vi "DB Tools Move To Next Record.vi"   [LabVIEW 2013, in "NI_Database_API_64.lvlib"]
doc: "Moves the cursor to point to the next record in the recordset identified by the reference. Wire data to the reference input to determine the polymorphic instance to use or manually select the instance."
uses:
  NI_Database_API_64.lvlib
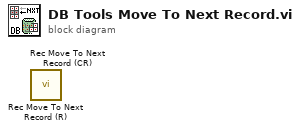
[diagram p0: block diagram]
diagram:
  n1 = call "Rec Move To Next Record (R).vi"() -> ()  [unwired: 10 in, 2 out]
  n2 = call "Rec Move To Next Record (CR).vi"() -> ()  [unwired: 10 in, 2 out]
